vi "Capacitance_IS_Test.vi"(7 "Published Data Id":T1, 9 "Frequencies":dbl[](array[numeric]), 10 "Data Id":string, 11 "Semiconductor Module Context":T2) -> (0 "error out":errorcluster)   [LabVIEW 2023, in "Capacitance.lvlib"]
doc: "Performs linear fitting on ZDut and extract Resonance Frequency and Capacitance values"
uses:
  Capacitance.lvlib
  <vilib>/NI_TestStand_SemiconductorModule/NI_TestStand_Semiconductor_Module.lvlibp/PinMap/General/SemiconductorModuleContext.ctl
  <vilib>/NI_TestStand_SemiconductorModule/NI_TestStand_Semiconductor_Module.lvlibp/PinMap/TagProvider/TSM_PublishedDataId.ctl
  <vilib>/NI_TestStand_SemiconductorModule/NI_TestStand_Semiconductor_Module.lvlibp/PinMap/General/Publish/PublishDataPerSiteDoubleScalar.vi
  <vilib>/NI_TestStand_SemiconductorModule/NI_TestStand_Semiconductor_Module.lvlibp
  <vilib>/Analysis/NI_AALPro.lvlib
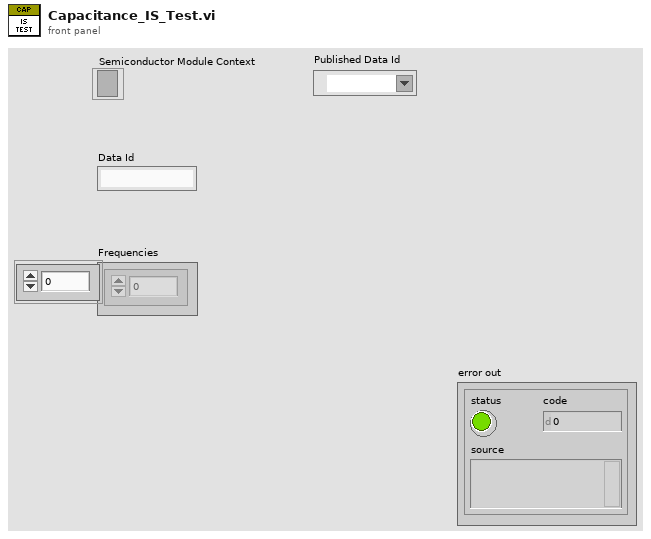
[diagram p1: front panel]
types:
  T1 = typedef "NI_TestStand_Semiconductor_Module.lvlibp/TSM_PublishedDataId.ctl" = tag
  T2 = typedef "NI_TestStand_Semiconductor_Module.lvlibp/SemiconductorModuleContext.ctl" = refnum<k7>
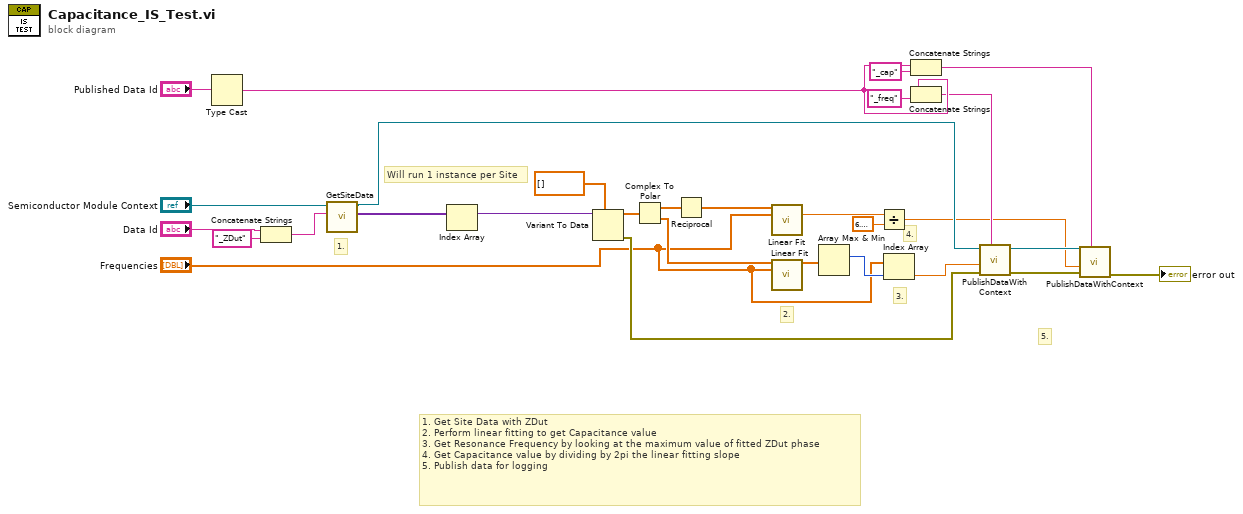
[diagram p0: block diagram]
diagram:
  # "4."
  # "3."
  # "2."
  # "Will run 1 instance per Site"
  # "1."
  # "1. Get Site Data with ZDut\n2. Perform linear fitting to get Capacitance value\n3. Get Resonance Frequency by looking at the maximum value of fitted ZDut phase\n4. Get Capacitance value by dividing by 2pi the linear fitting slope\n5. Publish data for logging"
  # "5."
  n1 = Type Cast(x="Published Data Id") -> (*(type *) &x=w19:string)  [unwired: 1 in]
  n2 = Concatenate Strings("Data Id", "_ZDut" ("string")) -> (w28:string)
  n3 = call <vilib>:"GetSiteData.vi"("Data Id"=w28, "Semiconductor Module Context"="Semiconductor Module Context") -> ("Site Data"=w27:variant[], "Semiconductor Module Context Out"=w22:T2)  [unwired: 7 in, 1 out]
  n4 = Index Array(array=w27) -> (element=w14:variant)  [unwired: 1 in]
  n5 = Variant To Data(type=cdb[] [], Variant=w14) -> (data=w11:cdb[], error out=w25:errorcluster)  [unwired: 1 in]
  n6 = Complex To Polar(r * e^(i*theta)=w11) -> (r=w10:dbl[], theta=w8:dbl[])
  n7 = Reciprocal(x=w10) -> (1/x=w9:dbl[])
  n8 = call <vilib>:"Linear Fit.vi"("Y"=w9, "X"="Frequencies") -> ("slope"=w4:dbl)  [unwired: 9 in, 4 out]
  n9 = call <vilib>:"Linear Fit.vi"("Y"=w8, "X"="Frequencies") -> ("Best Linear Fit"=w6:dbl[])  [unwired: 9 in, 4 out]
  n10 = Array Max & Min(array=w6) -> (max index (indices)=w7:i32)  [unwired: 3 out]
  n11 = Divide(x=w4, y=6.283185307179586) -> (x/y=w2:dbl)
  n12 = Index Array(array="Frequencies", index=w7) -> (element=w1:dbl)
  n13 = Concatenate Strings(w19, "_cap" ("string")) -> (w16:string)
  n14 = Concatenate Strings(w19, "_freq" ("string")) -> (w17:string)
  n15 = call-poly <vilib>:"PublishDataWithContext.vi"("Published Data Id"=w17, "error in (no error)"=w25, "Data In"=w1, "Semiconductor Module Context"=w22) -> ("error out"=w24:errorcluster, "Semiconductor Module Context Out"=w23:T2)  [unwired: 6 in]
  n16 = call-poly <vilib>:"PublishDataWithContext.vi"("Published Data Id"=w16, "error in (no error)"=w24, "Data In"=w2, "Semiconductor Module Context"=w23) -> ("error out"=→"error out":errorcluster)  [unwired: 6 in, 1 out]
